vi "DynamicModules.vi"() -> (3 "dynamic modules":string[](array[string]))   [LabVIEW 2017]
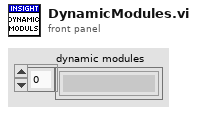
[diagram p1: front panel]
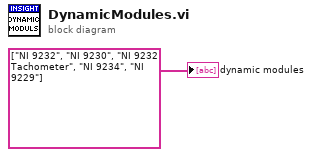
[diagram p0: block diagram]
diagram:
  "dynamic modules" <- string[] ["NI 9232", "NI 9230", "NI 9232 Tachometer", "NI 9234", "NI 9229"]
